vi "TrigConfig.vi"(4 "Trigger Level (V)":dbl, 6 "range (Vpp)":dbl, 8 "error in":errorcluster, 9 "Trigger Type":enum8{"Software", "Data Edge"}(ring), 10 "Requested Samples Per Pixel":u16, 11 "FPGA VI Reference":T1) -> (0 "error out":errorcluster, 2 "Read Size (Host)":u16, 3 "FPGA VI Reference Out":T1)   [LabVIEW 2020]
uses:
  DigiFPGARef.ctl
  <vilib>/Utility/error.llb/Error Cluster From Error Code.vi
  <vilib>/rvi/errors/niLvFpgaAdjustHostInterfaceError.vi
  <vilib>/rvi/interface/nirviReadWriteControl/nirviReadWriteControl.xnode
  NiFpgaLv.dll
  <vilib>/rvi/interface/Simulation/niFpgaSimulationCallBeginRW.vi
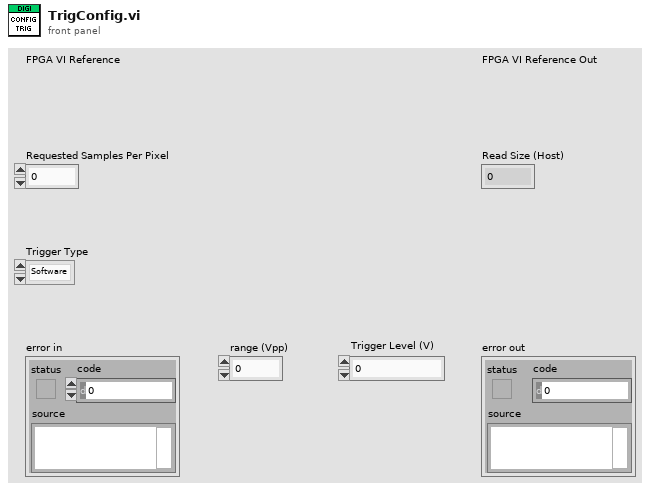
[diagram p1: front panel]
types:
  T1 = typedef "DigiFPGARef.ctl" = refnum<k20>
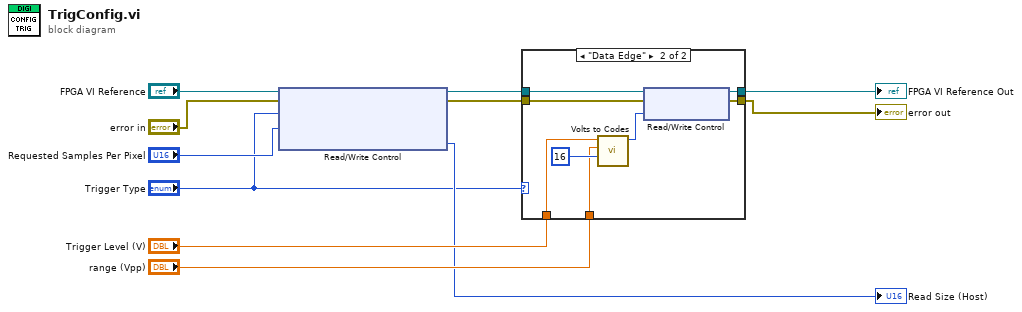
[diagram p0: block diagram]
diagram:
  n1 = xnode "Read/Write Control"("FPGA VI Reference In"="FPGA VI Reference", "error in"="error in", "Trigger Type"="Trigger Type", "Requested Samples Per Pixel"="Requested Samples Per Pixel") -> ("FPGA VI Reference Out"=w10:T1, "error out"=w11:errorcluster, "Read Size (Host)"=→"Read Size (Host)":u16)
  n2 = case shown="\"Data Edge\"" "Trigger Type" {
    tunnel: w10 -> [w13 w21]
    tunnel: w11 -> [w12 w20]
    tunnel: [w13 w19] -> w4
    tunnel: [w12 w18] -> w9
    tunnel: "range (Vpp)" -> [_ w15]
    tunnel: "Trigger Level (V)" -> [_ w14]
    frame "Software", Default {
    }
    frame "Data Edge" {
      n3 = call "Volts to Codes.vi"("Number of Bits"=i16 16, "range (Vpp)"=w15, "Data In"=w14) -> ("Data Out"=w16:i16)  [unwired: 8 out]
      n4 = xnode "Read/Write Control"("FPGA VI Reference In"=w21, "error in"=w20, "Trigger Level"=w16) -> ("FPGA VI Reference Out"=w19:T1, "error out"=w18:errorcluster)
    }
  }
  "error out" <- w9
  "FPGA VI Reference Out" <- w4
